vi "launch process ref bag.vi"(6 "launch items":T1, 7 "bag action":T2=enum."add", 11 "process ref IN":refnum<vi>) -> (1 "Keys":T1[](array[typedef]), 3 "process ref OUT":refnum<vi>)   [LabVIEW 2020]
uses:
  launch items list.ctl
  que event bag action.ctl
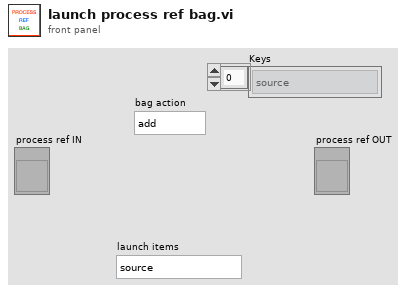
[diagram p1: front panel]
types:
  T1 = typedef "launch items list.ctl" = enum16{"source", "pll engine", "pll monitor", "sweeper engine", "sweeper monitor", "fitter"}
  T2 = typedef "que event bag action.ctl" = enum16{"check", "add", "init", "keys", "values"}
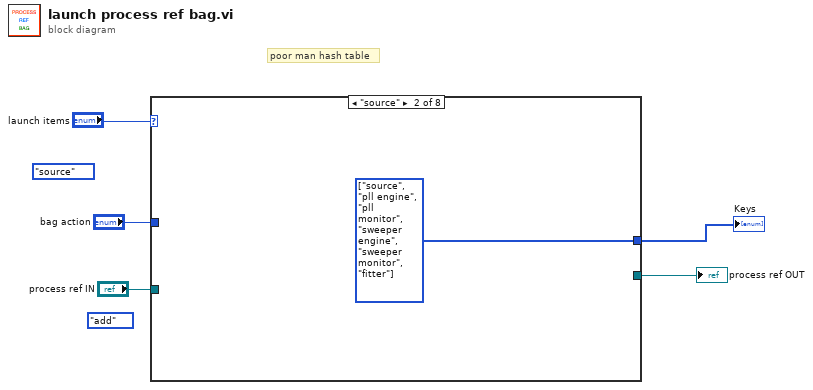
[diagram p0: block diagram]
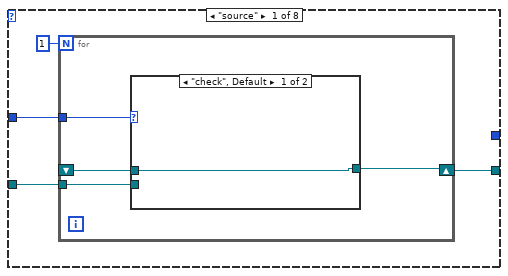
[diagram p2: hidden frame]
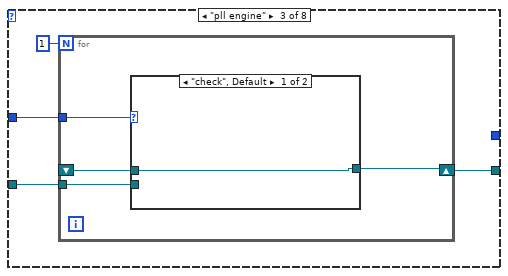
[diagram p4: hidden frame]
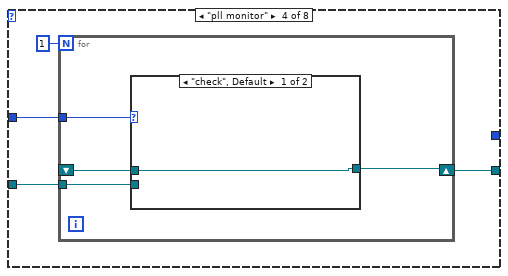
[diagram p6: hidden frame]
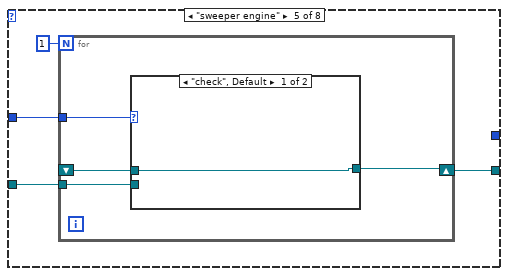
[diagram p8: hidden frame]
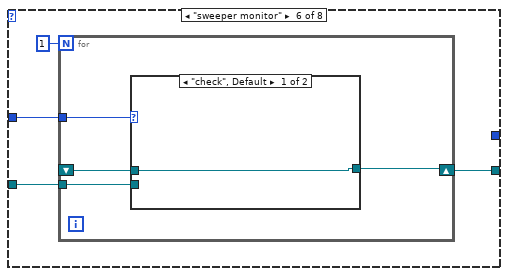
[diagram p10: hidden frame]
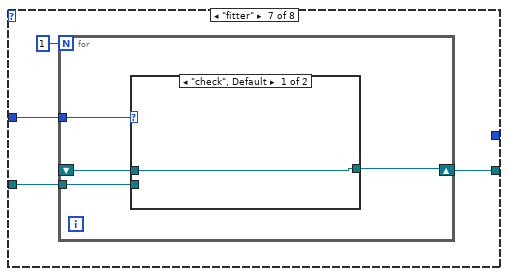
[diagram p12: hidden frame]
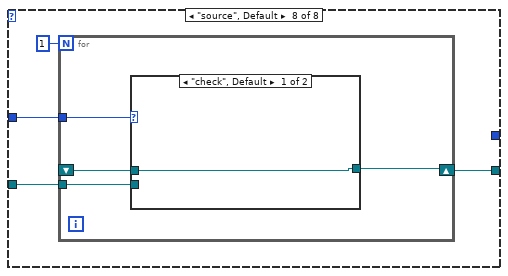
[diagram p14: hidden frame]
diagram:
  (unwired) que_event_bag_action."add" ("bag action")
  (unwired) launch_items_list."source" ("launch items")
  # "poor man hash table"
  n1 = case shown="\"--Keys\"" "launch items" {
    tunnel: "process ref IN" -> [w8 _ w19 w29 w39 w49 w59 w69]
    tunnel: "bag action" -> [w7 _ w18 w28 w38 w48 w58 w68]
    tunnel: [w6 _ w17 w27 w37 w47 w57 w67] -> w2
    tunnel: [_ w16 _ _ _ _ _ _] -> w1
    frame "source" {
      n2 = for {
        N: 1 -> [_]
        tunnel: w8 -> [w11]
        tunnel: w7 -> [w13]
        shift-right: [w12] -> w6
        shift-left: _ -> [w10]
        n3 = case shown="\"check\", Default" w13 {
          tunnel: [w14 w15] -> w12
          tunnel: w11 -> [_ w15]
          tunnel: w10 -> [w14 _]
          frame "check", Default {
          }
          frame "add" {
          }
        }
      }
    }
    frame "source" {
      w16 = T1[] [enum."source", enum."pll engine", enum."pll monitor", enum."sweeper engine", enum."sweeper monitor", enum."fitter"] items=["source", "pll engine", "pll monitor", "sweeper engine", "sweeper monitor", "fitter"]
    }
    frame "pll engine" {
      n4 = for {
        N: 1 -> [_]
        tunnel: w19 -> [w22]
        tunnel: w18 -> [w24]
        shift-right: [w23] -> w17
        shift-left: _ -> [w21]
        n5 = case shown="\"check\", Default" w24 {
          tunnel: [w25 w26] -> w23
          tunnel: w22 -> [_ w26]
          tunnel: w21 -> [w25 _]
          frame "check", Default {
          }
          frame "add" {
          }
        }
      }
    }
    frame "pll monitor" {
      n6 = for {
        N: 1 -> [_]
        tunnel: w29 -> [w32]
        tunnel: w28 -> [w34]
        shift-right: [w33] -> w27
        shift-left: _ -> [w31]
        n7 = case shown="\"check\", Default" w34 {
          tunnel: [w35 w36] -> w33
          tunnel: w32 -> [_ w36]
          tunnel: w31 -> [w35 _]
          frame "check", Default {
          }
          frame "add" {
          }
        }
      }
    }
    frame "sweeper engine" {
      n8 = for {
        N: 1 -> [_]
        tunnel: w39 -> [w42]
        tunnel: w38 -> [w44]
        shift-right: [w43] -> w37
        shift-left: _ -> [w41]
        n9 = case shown="\"check\", Default" w44 {
          tunnel: [w45 w46] -> w43
          tunnel: w42 -> [_ w46]
          tunnel: w41 -> [w45 _]
          frame "check", Default {
          }
          frame "add" {
          }
        }
      }
    }
    frame "sweeper monitor" {
      n10 = for {
        N: 1 -> [_]
        tunnel: w49 -> [w52]
        tunnel: w48 -> [w54]
        shift-right: [w53] -> w47
        shift-left: _ -> [w51]
        n11 = case shown="\"check\", Default" w54 {
          tunnel: [w55 w56] -> w53
          tunnel: w52 -> [_ w56]
          tunnel: w51 -> [w55 _]
          frame "check", Default {
          }
          frame "add" {
          }
        }
      }
    }
    frame "fitter" {
      n12 = for {
        N: 1 -> [_]
        tunnel: w59 -> [w62]
        tunnel: w58 -> [w64]
        shift-right: [w63] -> w57
        shift-left: _ -> [w61]
        n13 = case shown="\"check\", Default" w64 {
          tunnel: [w65 w66] -> w63
          tunnel: w62 -> [_ w66]
          tunnel: w61 -> [w65 _]
          frame "check", Default {
          }
          frame "add" {
          }
        }
      }
    }
    frame "source", Default {
      n14 = for {
        N: 1 -> [_]
        tunnel: w69 -> [w72]
        tunnel: w68 -> [w74]
        shift-right: [w73] -> w67
        shift-left: _ -> [w71]
        n15 = case shown="\"check\", Default" w74 {
          tunnel: [w75 w76] -> w73
          tunnel: w72 -> [_ w76]
          tunnel: w71 -> [w75 _]
          frame "check", Default {
          }
          frame "add" {
          }
        }
      }
    }
  }
  "process ref OUT" <- w2
  "Keys" <- w1
